vi "addClassToProject.vi"(8 "error in (no error)":errorcluster, 11 "targetClassPath":path) -> (0 "error out":errorcluster, 3 "classPath(dup)":path)   [LabVIEW 2023]
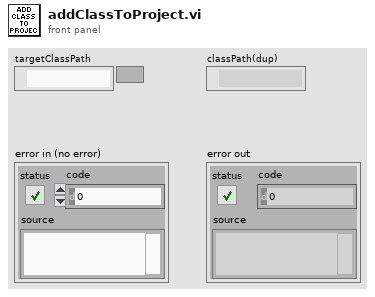
[diagram p1: front panel]
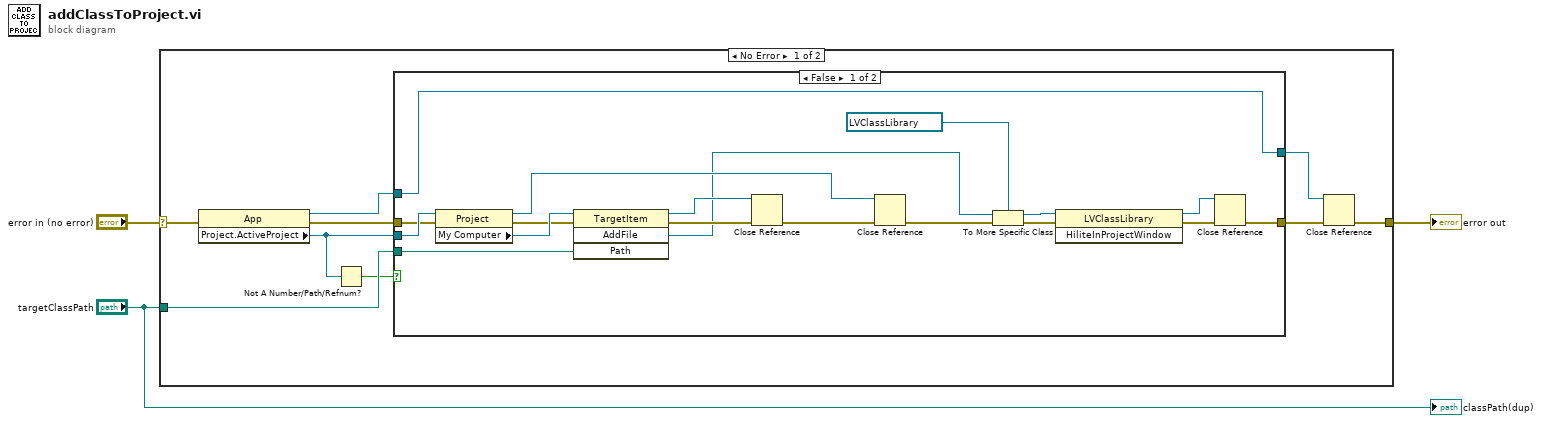
[diagram p0: block diagram]
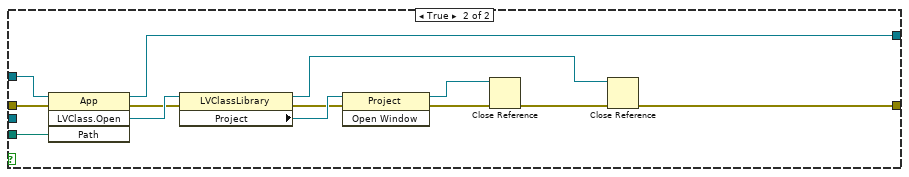
[diagram p2: hidden frame]
diagram:
  n1 = case shown="No Error" "error in (no error)" {
    selector: "error in (no error)" -> [w11 w44]
    tunnel: "targetClassPath" -> [w12 _]
    tunnel: [w4 w44] -> w2
    frame No Error {
      n2 = property class="App"(error in=w11) -> (reference out=w8:refnum<vi>, error out=w7:errorcluster, "Project.ActiveProject"=w6:refnum<vi>)  [unwired: 1 in]
      n3 = Not A Number/Path/Refnum?(number/path/refnum=w6) -> (NaN/Path/Refnum?=w5:bool)
      n4 = case shown="False" w5 {
        tunnel: w6 -> [w30 _]
        tunnel: w7 -> [w28 w34]
        tunnel: w12 -> [w22 w32]
        tunnel: [w17 w31] -> w10
        tunnel: w8 -> [w21 w35]
        tunnel: [w21 w33] -> w9
        frame False {
          n5 = property class="Project"(reference=w30, error in=w28) -> (reference out=w24:refnum<vi>, error out=w27:errorcluster, "My Computer"=w29:refnum<vi>)
          n6 = invoke class="TargetItem" method="AddFile"(reference=w29, error in=w27, "Path"=w22) -> (reference out=w25:refnum<vi>, error out=w26:errorcluster, "AddFile"=w13:refnum<vi>)  [unwired: 1 in, 1 out]
          n7 = Close Reference(reference=w25, error in (no error)=w26) -> (error out=w23:errorcluster)
          n8 = Close Reference(reference=w24, error in (no error)=w23) -> (error out=w20:errorcluster)
          n9 = To More Specific Class(target class=refnum<vi> refnum ("reference"), reference=w13, error in=w20) -> (specific class reference=w14:refnum<vi>, error out=w16:errorcluster)
          n10 = invoke class="LVClassLibrary" method="HiliteInProjectWindow"(reference=w14, error in=w16) -> (reference out=w18:refnum<vi>, error out=w19:errorcluster)  [unwired: 1 in, 1 out]
          n11 = Close Reference(reference=w18, error in (no error)=w19) -> (error out=w17:errorcluster)
        }
        frame True {
          n12 = invoke class="App" method="LVClass.Open"(reference=w35, error in=w34, "Path"=w32) -> (reference out=w33:refnum<vi>, error out=w42:errorcluster, "LVClass.Open"=w43:refnum<vi>)  [unwired: 1 in, 1 out]
          n13 = property class="LVClassLibrary"(reference=w43, error in=w42) -> (reference out=w41:refnum<vi>, error out=w39:errorcluster, "Project"=w40:refnum<vi>)
          n14 = invoke class="Project" method="Open Window"(reference=w40, error in=w39) -> (reference out=w38:refnum<vi>, error out=w37:errorcluster)  [unwired: 1 in, 1 out]
          n15 = Close Reference(reference=w38, error in (no error)=w37) -> (error out=w36:errorcluster)
          n16 = Close Reference(reference=w41, error in (no error)=w36) -> (error out=w31:errorcluster)
        }
      }
      n17 = Close Reference(reference=w9, error in (no error)=w10) -> (error out=w4:errorcluster)
    }
    frame Error {
    }
  }
  "error out" <- w2
  "classPath(dup)" <- "targetClassPath"
